vi "Teleop.vi"(10 "Match Info":T1={"Autonomous Elapsed Seconds"=0.0, "TeleOp Elapsed Seconds"=0.0, "Disabled Elapsed Seconds"=0.0, "Visited Autonomous"=FALSE, "Visited TeleOp"=FALSE, "Visited Disabled"=FALSE, "Autonomous Settings"={"Autonomous Style"=enum."Independent", "VI Refnum"=refnum}}, 11 "Call Context":T2) -> ()   [LabVIEW 2016]
doc: "This VI is called for each TeleOp packet received from the DS where the robot is not disabled. It is often used to read from the joysticks and update I/O or to update setpoints for timed control loops. It should complete and return within 20 milliseconds or it may miss DS packets."
uses:
  <vilib>/Rock Robotics/WPI/DriverStation/WPI_DriverStationDerivedRobotMode.ctl
  <vilib>/Rock Robotics/WPI/DriverStation/WPI_DriverStationMatch Info.ctl
  <vilib>/Rock Robotics/Network Tables/NT Read Boolean.vi
  <vilib>/Rock Robotics/Network Tables/NT Read Number.vi
  <vilib>/Rock Robotics/WPI/Utilities/WPI_GetSetVariantRefNum.vi
  Globals/Joystick1_YAxis.vi
  Globals/Joystick2_YAxis.vi
  Globals/WindowMotorValue.vi
  Globals/SpinnerMotorsValue.vi
panel:
  out "Sample Slider 0":dbl(slide) scale=0.0..5.0
  out "Sample Boolean 1":bool
  out "Sample Boolean 0":bool
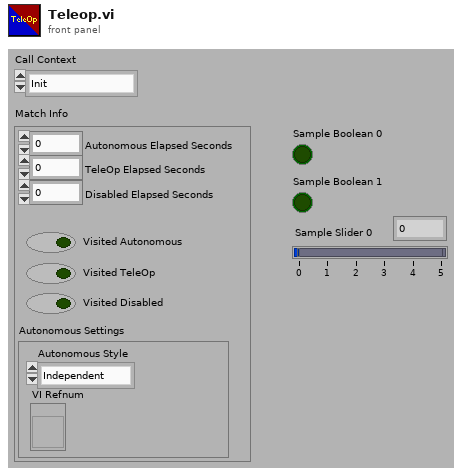
[diagram p1: front panel]
types:
  T1 = typedef "WPI_DriverStationMatch Info.ctl" = cluster{"Autonomous Elapsed Seconds":dbl, "TeleOp Elapsed Seconds":dbl, "Disabled Elapsed Seconds":dbl, "Visited Autonomous":bool, "Visited TeleOp":bool, "Visited Disabled":bool, "Autonomous Settings":cluster{"Autonomous Style":enum16{"Iterative", "Independent"}, "VI Refnum":refnum<vi>}}
  T2 = typedef "WPI_DriverStationDerivedRobotMode.ctl" = enum16{"Init", "Execute", "Stop"}
  T3 = typedef "WPI_JoystickDevRef.ctl" = cluster{"Device":T4}
  T4 = typedef "WPI_JoystickDeviceEnum.ctl" = enum16{"USB 0", "USB 1", "USB 2", "USB 3", "USB 4", "USB 5"}
  T5 = cluster{"Axes[0]":dbl, "Axes[1]":dbl, "Axes[2]":dbl, "Axes[3]":dbl, "Axes[4]":dbl, "Axes[5]":dbl, "Axes[6]":dbl, "Axes[7]":dbl, "Axes[8]":dbl}
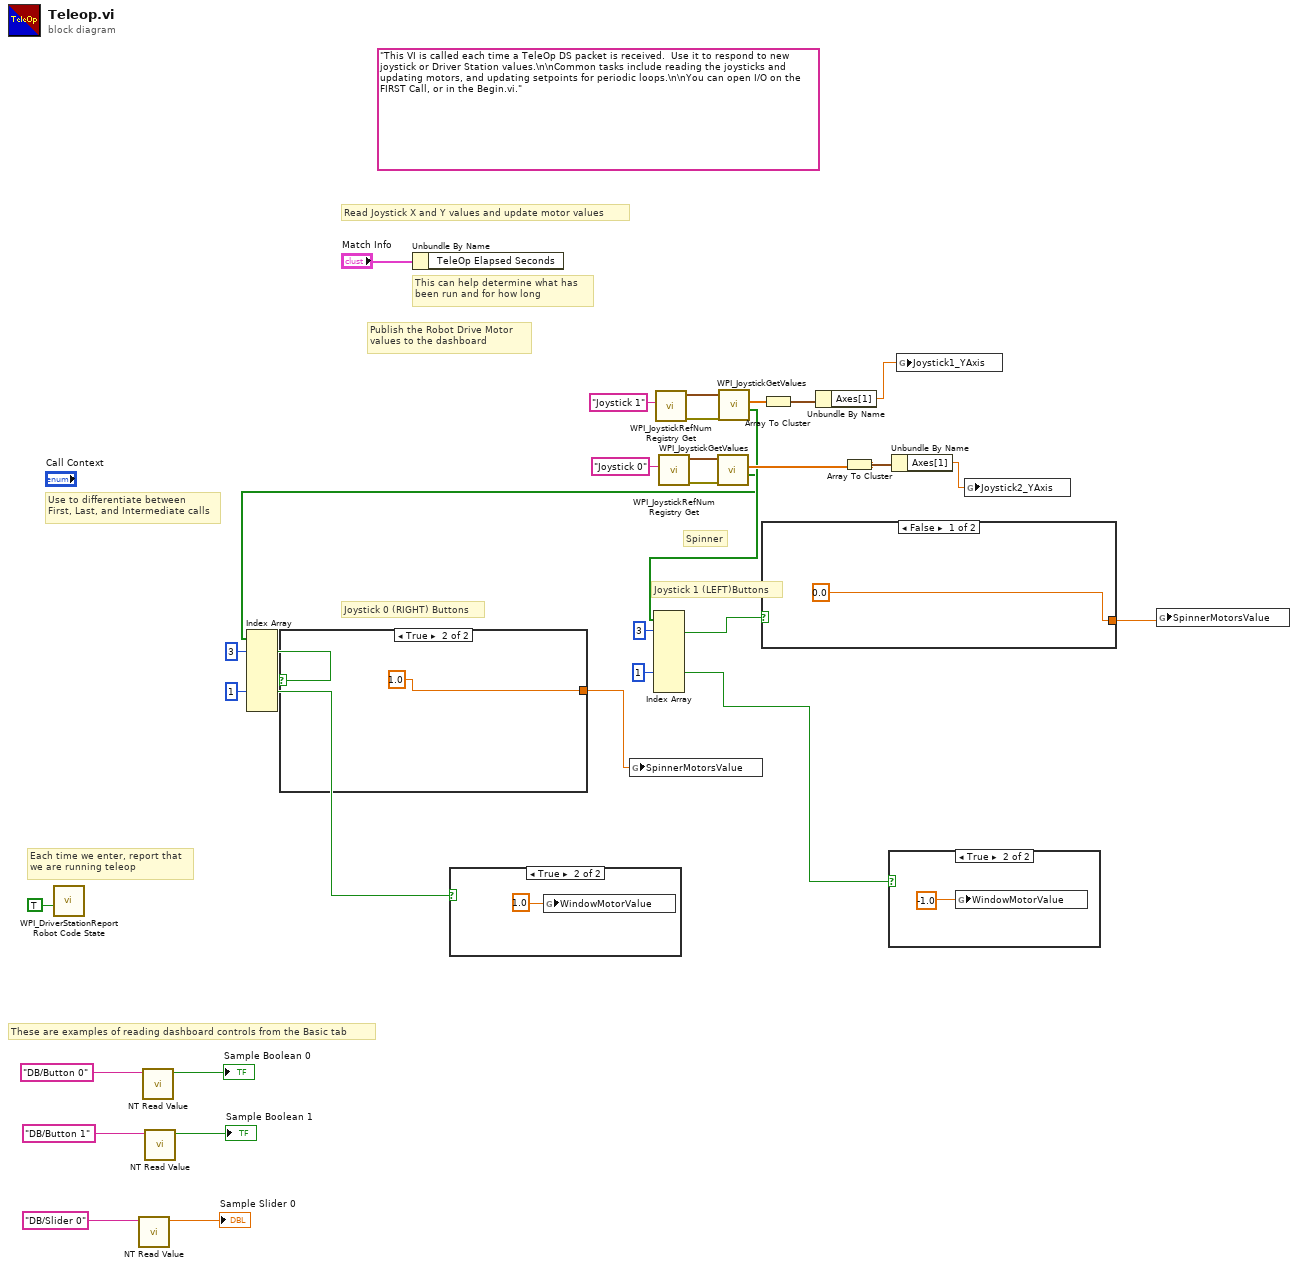
[diagram p0: block diagram]
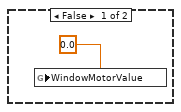
[diagram p2: hidden frame]
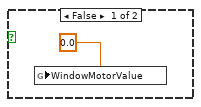
[diagram p3: hidden frame]
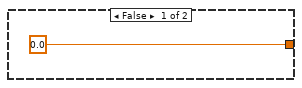
[diagram p4: hidden frame]
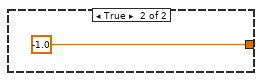
[diagram p5: hidden frame]
diagram:
  (unwired) "This VI is called each time a TeleOp DS packet is received.  Use it to respond to new joystick or Driver Station values.\n\nCommon tasks include reading the joysticks and updating motors, and updating setpoints for periodic loops.\n\nYou can open I/O on the FIRST Call, or in the Begin.vi."
  # "Joystick 1 (LEFT)Buttons"
  # "Joystick 0 (RIGHT) Buttons"
  # "Spinner"
  # "These are examples of reading dashboard controls from the Basic tab"
  # "Publish the Robot Drive Motor\nvalues to the dashboard"
  # "Each time we enter, report that\nwe are running teleop"
  # "Use to differentiate between\nFirst, Last, and Intermediate calls"
  # "This can help determine what has\nbeen run and for how long"
  # "Read Joystick X and Y values and update motor values"
  n1 = call <vilib>:"WPI_DriverStationReport Robot Code State.vi"("TeleOp"=TRUE ("Autonomous")) -> ()  [unwired: 10 in, 1 out]
  n2 = call-poly <vilib>:"NT Read Value.vi"("Name"="DB/Slider 0" ("refnum name")) -> ("Numeric"=→"Sample Slider 0":dbl)  [unwired: 9 in, 1 out]
  n3 = call-poly <vilib>:"NT Read Value.vi"("Name"="DB/Button 0" ("refnum name")) -> ("Boolean"=→"Sample Boolean 0":bool)  [unwired: 9 in, 1 out]
  n4 = call-poly <vilib>:"NT Read Value.vi"("Name"="DB/Button 1" ("refnum name")) -> ("Boolean"=→"Sample Boolean 1":bool)  [unwired: 9 in, 1 out]
  n5 = Unbundle By Name("Match Info") -> ()  [unwired: 1 out]
  n6 = call <vilib>:"WPI_JoystickRefNum Registry Get.vi"("refnum name"="Joystick 1") -> ("error out"=w5:errorcluster, "JoystickDevRef"=w24:T3)  [unwired: 9 in]
  n7 = call <vilib>:"WPI_JoystickRefNum Registry Get.vi"("refnum name"="Joystick 0") -> ("error out"=w6:errorcluster, "JoystickDevRef"=w23:T3)  [unwired: 9 in]
  n8 = call <vilib>:"WPI_JoystickGetValues.vi"("error in (no error)"=w6, "JoystickDevRef"=w23) -> ("Buttons"=w11:bool[], "Axes"=w17:dbl[])  [unwired: 5 in, 3 out]
  n9 = Index Array(array=w11, index #1=3 ("index"), index #6=1 ("index")) -> (element #1=w13:bool, element #6=w7:bool)  [unwired: 6 in, 6 out]
  n10 = case shown="True" w13 {
    tunnel: [0.0 ("Output") 1.0 ("Output")] -> w2
    frame False {
    }
    frame True {
    }
  }
  n11 = case shown="True" w7 {
    frame False {
      n12 = global write "WindowMotorValue.vi" "WindowMotorValue"(0.0 ("Output")) -> ()
    }
    frame True {
      n13 = global write "WindowMotorValue.vi" "WindowMotorValue"(1.0 ("Output")) -> ()
    }
  }
  n14 = global write "SpinnerMotorsValue.vi" "SpinnerMotorsValue"(w2) -> ()
  n15 = call <vilib>:"WPI_JoystickGetValues.vi"("error in (no error)"=w5, "JoystickDevRef"=w24) -> ("Buttons"=w12:bool[], "Axes"=w20:dbl[])  [unwired: 5 in, 3 out]
  n16 = Index Array(array=w12, index #1=3 ("index"), index #6=1 ("index")) -> (element #1=w16:bool, element #6=w8:bool)  [unwired: 6 in, 6 out]
  n17 = case shown="False" w16 {
    tunnel: [0.0 ("Output") -1.0 ("Output")] -> w1
    frame False {
    }
    frame True {
    }
  }
  n18 = Array To Cluster(array=w20) -> (cluster=w19:T5)
  n19 = Unbundle By Name(w19) -> ("Axes[1]"=w4:dbl)
  n20 = Array To Cluster(array=w17) -> (cluster=w18:T5)
  n21 = case shown="True" w8 {
    frame False {
      n22 = global write "WindowMotorValue.vi" "WindowMotorValue"(0.0 ("Output")) -> ()
    }
    frame True {
      n23 = global write "WindowMotorValue.vi" "WindowMotorValue"(-1.0 ("Output")) -> ()
    }
  }
  n24 = Unbundle By Name(w18) -> ("Axes[1]"=w3:dbl)
  n25 = global write "Joystick1_YAxis.vi" "Joystick1_YAxis"(w4) -> ()
  n26 = global write "Joystick2_YAxis.vi" "Joystick2_YAxis"(w3) -> ()
  n27 = global write "SpinnerMotorsValue.vi" "SpinnerMotorsValue"(w1) -> ()
